vi "Get Constant.vi"(1 "Selection":T1) -> (0 "String":string)   [LabVIEW 2019, in "gRPC Template Creation Utility.lvlib"]
uses:
  gRPC Template Creation Utility.lvlib
  OneOfConstantsEnum.ctl
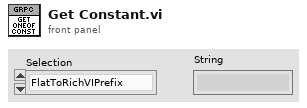
[diagram p1: front panel]
types:
  T1 = typedef "gRPC Template Creation Utility.lvlib/OneOfConstantsEnum.ctl" = enum16{"FlatToRichVIPrefix", "RichToFlatVIPrefix", "FlatTypeDefSuffix"}
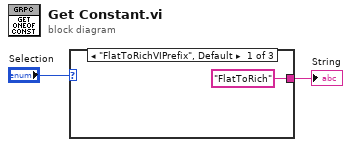
[diagram p0: block diagram]
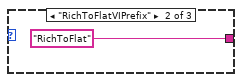
[diagram p2: hidden frame]
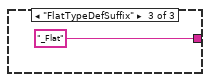
[diagram p3: hidden frame]
diagram:
  n1 = case shown="\"FlatToRichVIPrefix\", Default" "Selection" {
    tunnel: ["FlatToRich" "RichToFlat" "_Flat"] -> w1
    frame "FlatToRichVIPrefix", Default {
    }
    frame "RichToFlatVIPrefix" {
    }
    frame "FlatTypeDefSuffix" {
    }
  }
  "String" <- w1
